vi "Reorder 1D Array of funct data.vi"(9 "indices":i32[](array[numeric]), 11 "Data in":T1) -> (3 "Data out":T1)   [LabVIEW 2017]
doc: "This polymorphic VI reorders a 1D or 2D <B>array</B> of any size based on the indices you specify. For 2D arrays, it reorders by row or by column."
uses:
  xcontrol/Interface VIs/Interface typedefs/Interface-Data array.ctl
  xcontrol/Interface VIs/Interface typedefs/Interface-Data format definition.ctl
  xcontrol/Typedefs/Xctl-XY data type definition.ctl
  xcontrol/Typedefs/Xctrl-ROI type enum.ctl
  xcontrol/XGrapher.xctl
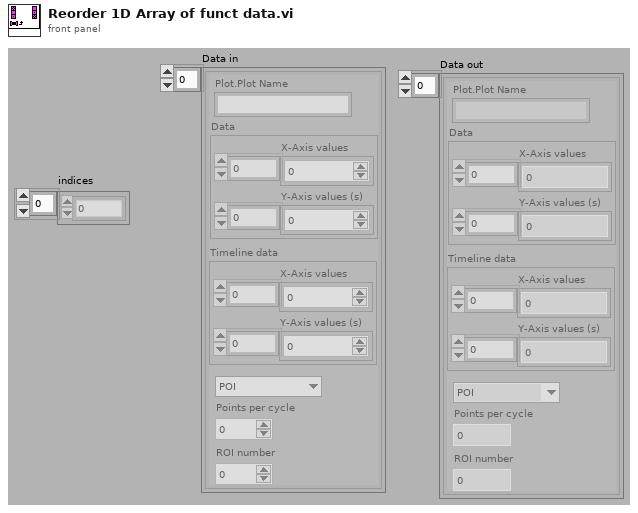
[diagram p1: front panel]
types:
  T1 = typedef "Interface-Data array.ctl" = T2[]
  T2 = typedef "Interface-Data format definition.ctl" = cluster{"Plot.Plot Name":string, "Data":T3, "Timeline data":T3, "Type":T4, "Points per cycle":u16, "ROI number":u16}
  T3 = typedef "XGrapher.xctl/Xctl-XY data type definition.ctl" = cluster{"X-Axis values":sgl[], "Y-Axis values (s)":sgl[]}
  T4 = typedef "Xctrl-ROI type enum.ctl" = enum16{"POI", "Mini-scan", "Group"}
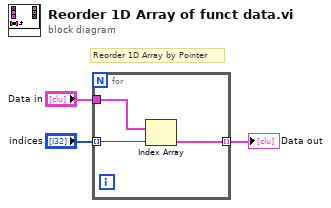
[diagram p0: block diagram]
diagram:
  # "Reorder 1D Array by Pointer"
  n1 = for {
    tunnel: "Data in" -> [w6]
    tunnel: [w5] -> w2 mode=indexing
    tunnel: "indices" -> [w4] mode=indexing
    n2 = Index Array(array=w6, index=w4) -> (element=w5:T2)
  }
  "Data out" <- w2
